vi "DT 3 Cells.vi"(0 "DT 3 Cells":i32[](array[numeric]), 5 "Count":i32[](array[numeric]), 11 "error in (no error)":errorcluster) -> (4 "DT 3 Cells":i32[](array[numeric]), 6 "# of DT 3 Cells":i32, 15 "error out":errorcluster)   [LabVIEW 2014]
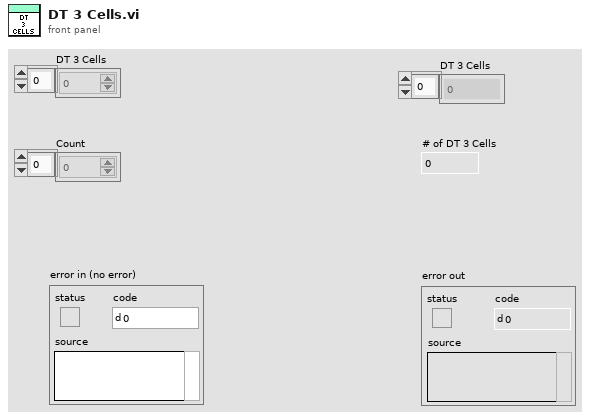
[diagram p1: front panel]
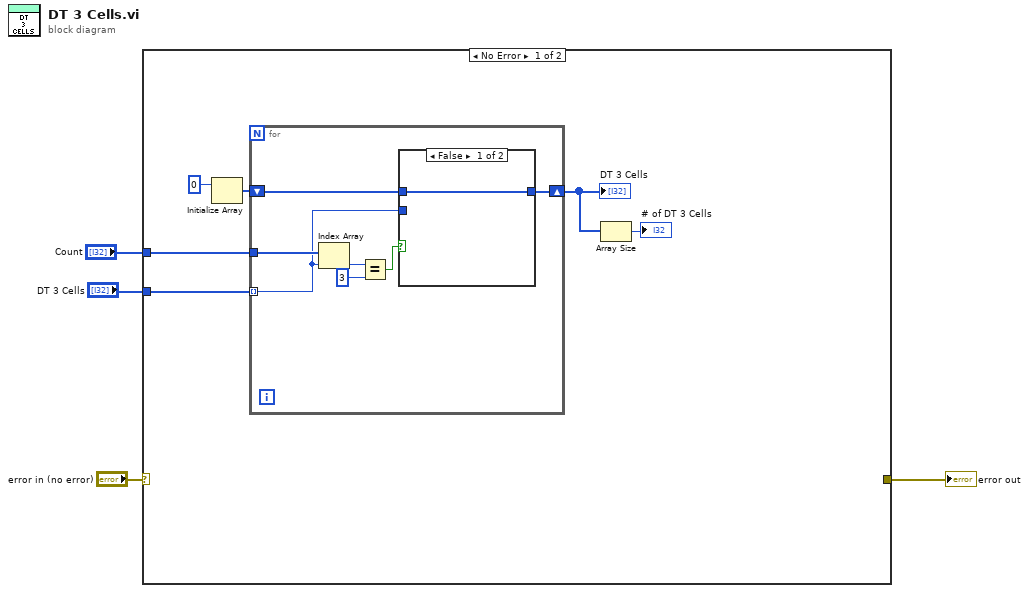
[diagram p0: block diagram]
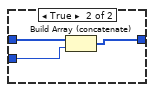
[diagram p2: hidden frame]
diagram:
  n1 = case shown="No Error" "error in (no error)" {
    selector: "error in (no error)" -> [_ w22]
    tunnel: [_ w22] -> w3
    tunnel: "DT 3 Cells" -> [w10 _]
    tunnel: "Count" -> [w9 _]
    frame No Error {
      n2 = Initialize Array(0) -> (w8:i32[])  [unwired: 1 in]
      n3 = for {
        tunnel: w10 -> [w12] mode=indexing
        tunnel: w9 -> [w17]
        shift-right: [w11] -> w6
        shift-left: w8 -> [w13]
        n4 = Index Array(array=w17, index=w12) -> (element=w16:i32)
        n5 = Equal?(x=w16, y=3) -> (x = y?=w14:bool)
        n6 = case shown="False" w14 {
          tunnel: w13 -> [w18 w21]
          tunnel: w12 -> [_ w20]
          tunnel: [w18 w19] -> w11
          frame False {
          }
          frame True {
            n7 = Build Array (concatenate)(w21, w20) -> (w19:i32[])
          }
        }
      }
      "DT 3 Cells" <- w6
      n8 = Array Size(array=w6) -> (size(s)=→"# of DT 3 Cells":i32)
    }
    frame Error {
    }
  }
  "error out" <- w3
